vi "Timestamp to Unix epoch time.vi"(10 "Precision (ms)":T1=enum."milliseconds", 11 "Timestamp":timestamp format="%<%I:%M:%S%3u %p\n%Y/%m/%d>T") -> (3 "Unix epoch time":u64)   [LabVIEW 2015, in "InfluxDB Client.lvclass"]
doc: "Convert the LabVIEW timestamp format to Unix epoch time."
uses:
  InfluxDB Client.lvclass
  Time precision.ctl
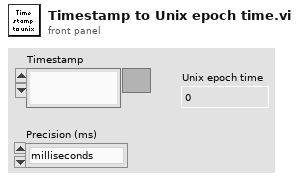
[diagram p1: front panel]
types:
  T1 = typedef "InfluxDB Client.lvclass/Time precision.ctl" = enum16{"seconds", "milliseconds", "microseconds"}
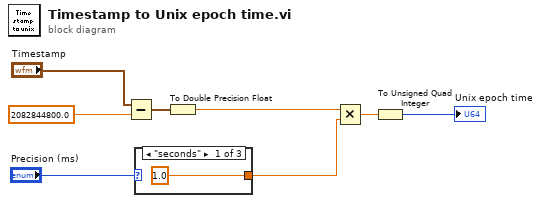
[diagram p0: block diagram]
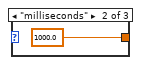
[diagram p2: hidden frame]
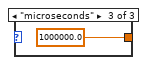
[diagram p3: hidden frame]
diagram:
  n1 = Subtract(x="Timestamp", y=2082844800.0) -> (x-y=w4:timestamp)
  n2 = case shown="\"seconds\"" "Precision (ms)" {
    tunnel: [1.0 ("Database name") 1000.0 ("Database name") 1000000.0 ("Database name")] -> w1
    frame "seconds" {
    }
    frame "milliseconds" {
    }
    frame "microseconds" {
    }
  }
  n3 = To Double Precision Float(number=w4) -> (double precision float=w6:dbl)
  n4 = Multiply(x=w6, y=w1) -> (x*y=w5:dbl)
  n5 = To Unsigned Quad Integer(1:w5) -> (0:→"Unix epoch time":u64)
